vi "3D_Traverse_move.vi"(0 "Mode":T4=enum."Read traverse position", 1 "Route Checking?":bool=TRUE, 2 "Row Number":i32=-1, 5 "Position":sgl[](array[numeric])=[0.0, 0.0, 0.0] format="%#.2f", 7 "Work in Tunnel Coordinates":T2, 9 "Home":T1, 11 "Simulate/Run":T3=enum."Run VI", 12 "Traverse name":string, 13 "Backlash Compensation?":bool=TRUE, 14 "Currently on Point":i32=-1) -> (3 "Model  Roll        Pitch       Yaw (deg)":sgl[](array[numeric]) format="%#.2f", 4 "Trav Position achieved":sgl[](array[numeric]) format="%#.2f", 15 "Error String":string)   [LabVIEW 2014]
uses:
  Trav_mode.ctl
  Controls/User_Specific_mode.ctl
  Controls/Tunnel_Coordinates.ctl
  Controls/Home.ctl
  Controls/Global_mode.ctl
  Route mapping/Route_Display_Mode.ctl
  ADAM Client/Sub VIs/ADAM Controls/Update_scan_value.ctl
  Controls/In_Range.ctl
  Globals/Trav_pos_global.vi
  Globals/Preference_global.vi
  Globals/Constants_global.vi
  Route mapping/Route_mapping_global.vi
panel:
  in  "Position Increment":sgl[](array[numeric])=[0.0, 0.0, 0.0] step=1 format="%#.2f"
  out "Traverses Available":string[](array[string])
  in  "Traverse":u16(ring) items=["EnFlo_Measure_Height", "EnFlo_Stack", "EnFlo_Stack  dfg", "EnFlo_Trav3", "EnFlo_Tunnel", "EnFlo_Turntable"]
  # "X                Y                   Z"
  # "X                Y                   Z"
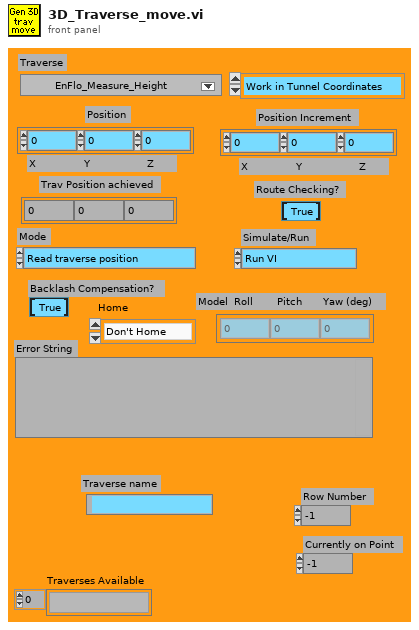
[diagram p1: front panel]
types:
  T1 = typedef "Home.ctl" = enum16{"Don't Home", "Home  +X", "Home  -X", "Home  +Y", "Home  -Y", "Home  +Z", "Home  -Z"}
  T2 = typedef "Tunnel_Coordinates.ctl" = enum16{"Work in Tunnel Coordinates", "Work in Model Coordinates"}
  T3 = typedef "User_Specific_mode.ctl" = enum16{"Check VI only", "Run VI"}
  T4 = typedef "Trav_mode.ctl" = enum16{"Move traverse", "Read traverse position", "Teach Position"}
  T5 = typedef "Global_mode.ctl" = enum16{"Read Global", "Load Global From File", "Write Global to File"}
  T6 = enum16{"To Traverse Coordinates", "To User Coordinates"}
  T7 = typedef "Route_Display_Mode.ctl" = enum16{"Display View Always", "Display View on Crash"}
  T8 = typedef "Update_scan_value.ctl" = cluster{"Channel Name":string, "New Value":dbl}
  T9 = typedef "In_Range.ctl" = enum16{"%", "±", "% & ±"}
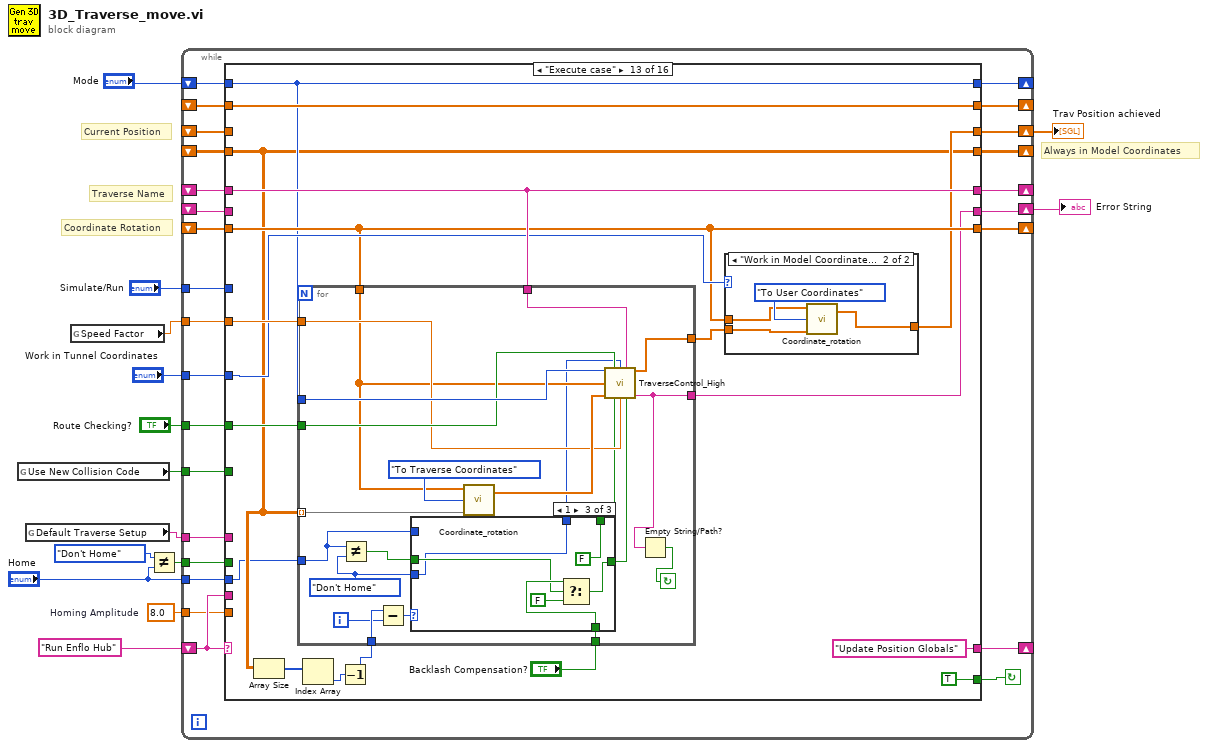
[diagram p0: block diagram]
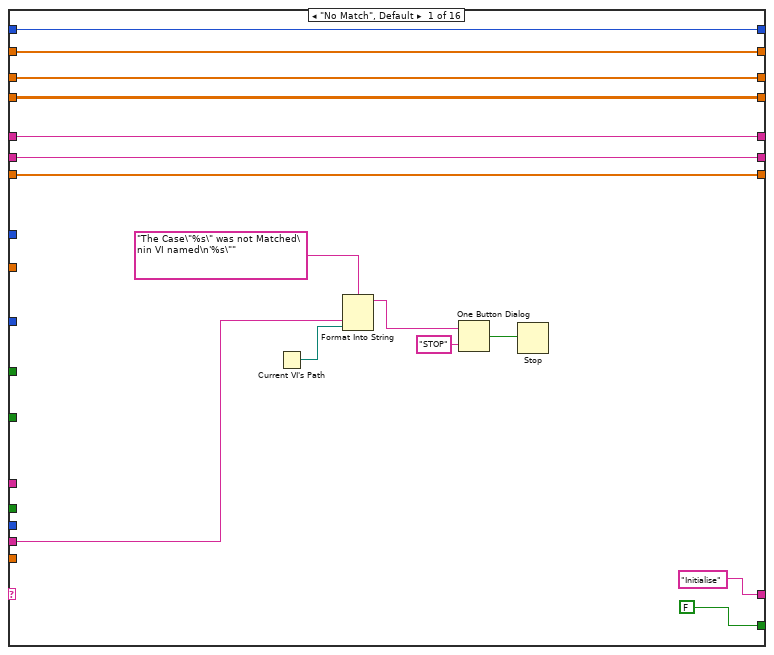
[diagram p2: hidden frame]
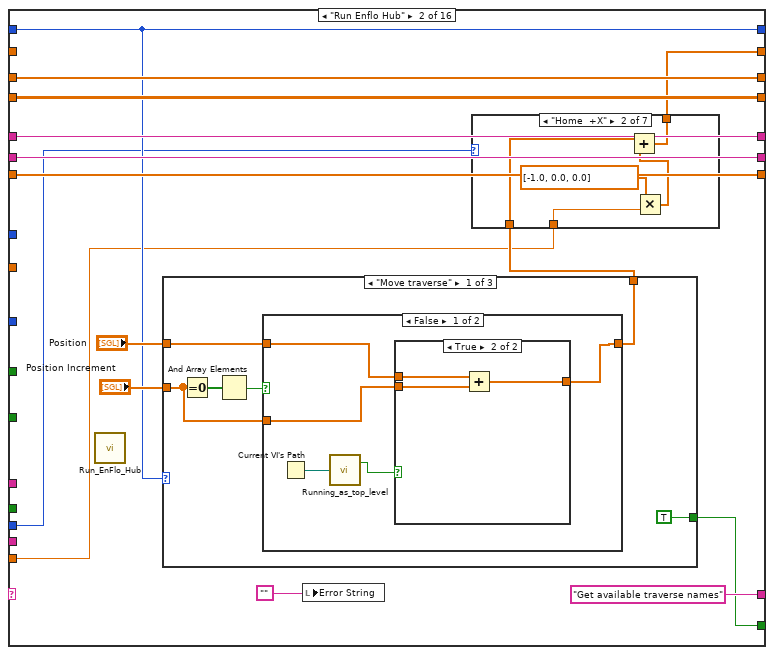
[diagram p3: hidden frame]
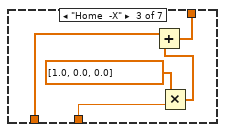
[diagram p5: hidden frame]
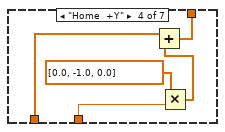
[diagram p6: hidden frame]
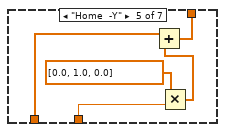
[diagram p7: hidden frame]
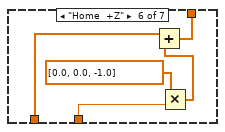
[diagram p8: hidden frame]
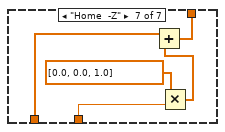
[diagram p9: hidden frame]
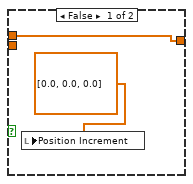
[diagram p10: hidden frame]
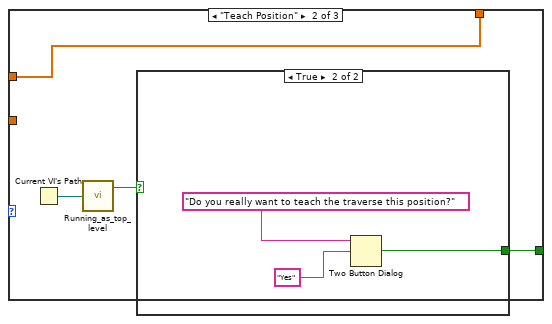
[diagram p12: hidden frame]
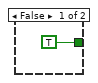
[diagram p13: hidden frame]
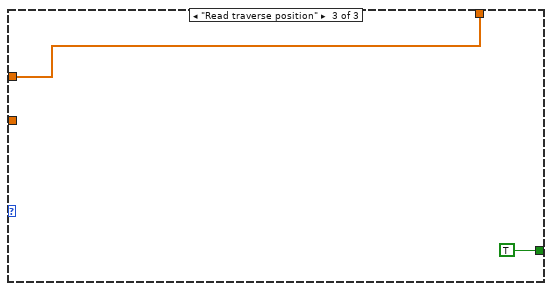
[diagram p14: hidden frame]
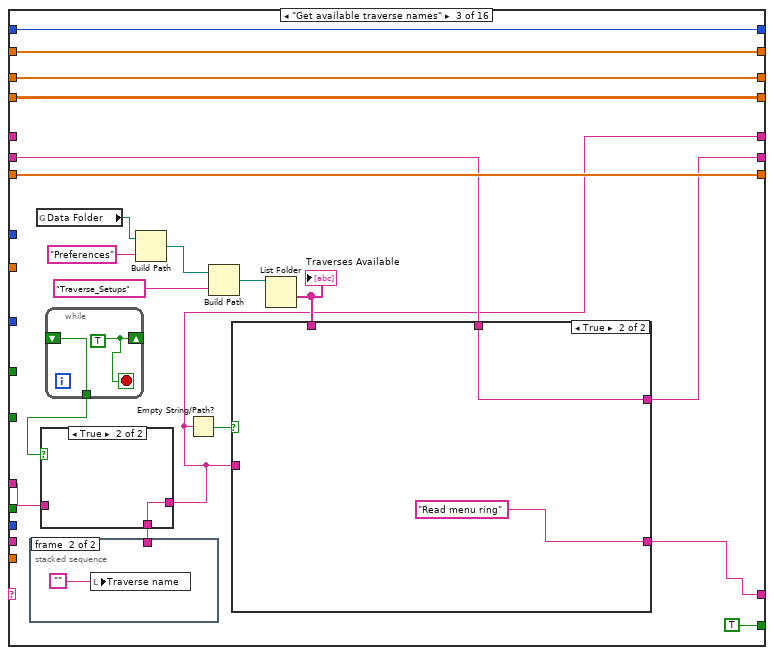
[diagram p15: hidden frame]
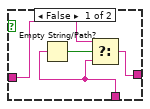
[diagram p16: hidden frame]
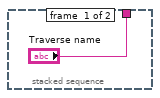
[diagram p17: hidden frame]
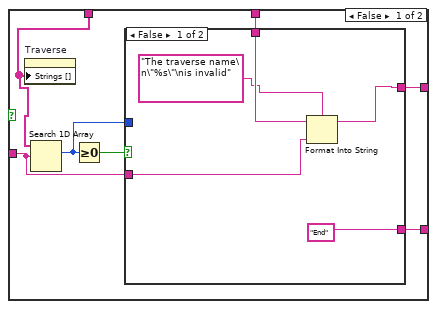
[diagram p18: hidden frame]
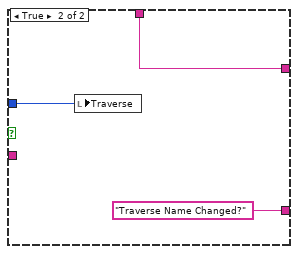
[diagram p19: hidden frame]
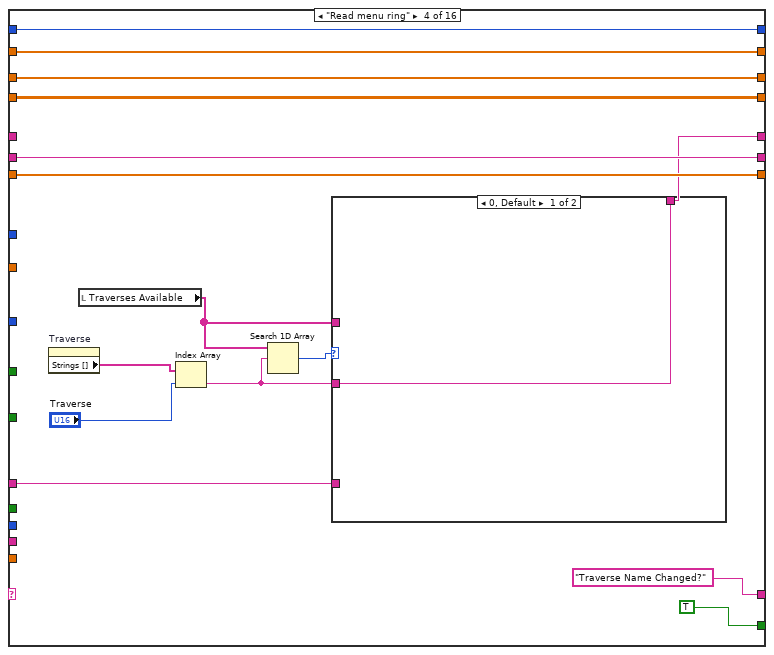
[diagram p20: hidden frame]
diagram:
  w5 = sgl 8.0  # Homing Amplitude
  # "Always in Model Coordinates"
  # "Current Position"
  # "Coordinate Rotation"
  # "Traverse Name"
  n1 = global read "Preference_global.vi" "Use New Collision Code"() -> (w1:bool)
  n2 = global read "Trav_pos_global.vi" "Default Traverse Setup"() -> (w7:string)
  n3 = global read "Trav_pos_global.vi" "Speed Factor"() -> (w11:sgl)
  n4 = Not Equal?(x=Home."Don't Home" ("Home"), y="Home") -> (x != y?=w2:bool)
  n5 = while {
    shift-left: "Run Enflo Hub" -> [w38]
    shift-right: [w39] -> _
    shift-right: [w36] -> _
    shift-left: _ -> [w34]
    tunnel: "Simulate/Run" -> [w37]
    shift-right: [w35] -> w12
    shift-left: _ -> [w33]
    shift-right: [w31] -> _
    shift-left: _ -> [w32]
    shift-right: [w28] -> _
    shift-left: _ -> [w27]
    shift-right: [w29] -> w8
    shift-left: _ -> [w30]
    tunnel: w11 -> [w26]
    tunnel: "Work in Tunnel Coordinates" -> [w25]
    tunnel: "Route Checking?" -> [w24]
    tunnel: w7 -> [w23]
    shift-right: [w22] -> _
    shift-left: _ -> [w21]
    shift-right: [w19] -> _
    shift-left: "Mode" -> [w20]
    tunnel: "Home" -> [w18]
    tunnel: w5 -> [w17]
    tunnel: w2 -> [w16]
    tunnel: w1 -> [w15]
    stop <- w40 continue-if-true
    n6 = case shown="\"Execute case\"" w38 {
      tunnel: [FALSE w63 TRUE TRUE TRUE TRUE w311 TRUE ("T button?") TRUE ("T button?") TRUE w503 w531 TRUE TRUE TRUE FALSE] -> w40
      tunnel: ["Initialise" "Get available traverse names" w139 "Traverse Name Changed?" "Mode" w261 w301 "Perform Route Check" w361 w403 "Display Traverse Views" w538 "Update Position Globals" "Tidy up" "End" "End"] -> w39
      tunnel: w38 -> [w50 _ _ _ _ _ _ _ _ _ _ _ _ _ _ _]
      tunnel: w37 -> [_ _ _ _ w214 w262 w306 _ w358 w399 _ w536 _ w626 w679 w776]
      tunnel: [w47 w69 w131 w175 w207 w253 w313 w338 w360 w398 w508 w543 w580 w625 w684 w772] -> w36
      tunnel: [w46 w68 w137 w187 "" w263 w312 "" w353 w407 w500 w540 w564 w629 w686 w779] -> w35
      tunnel: w34 -> [w47 w69 _ _ w207 w253 w313 w338 w360 w398 w508 w543 w580 w625 w684 w772]
      tunnel: w33 -> [w46 w68 w136 w187 _ w263 _ _ w355 _ w501 w540 _ w629 w687 w779]
      tunnel: w32 -> [w45 w67 w148 w186 _ w264 w309 w341 w356 w390 w496 w546 w577 w622 w689 w773]
      tunnel: [w45 w67 w148 w186 w206 w264 w309 w341 w356 w390 w496 w546 w577 w622 w689 w773] -> w31
      tunnel: w30 -> [w44 w66 w147 w185 w217 w255 w307 _ w352 w405 w507 w545 _ w624 w688 w774]
      tunnel: [w44 w66 w147 w185 w217 w255 w299 w340 w352 w406 w507 w545 w575 w624 w688 w774] -> w29
      tunnel: [w43 w65 w146 w184 w218 w265 w314 w344 w365 w393 w506 w544 w569 w630 w690 w780] -> w28
      tunnel: w27 -> [w43 w65 w146 w184 _ w265 w314 w344 w365 _ w506 w544 w569 w630 w690 w780]
      tunnel: w26 -> [_ _ _ _ _ _ _ _ _ _ _ _ w579 _ _ _]
      tunnel: w25 -> [_ _ _ _ w213 w257 w310 w342 w357 w408 w497 _ w578 w623 _ w775]
      tunnel: w24 -> [_ _ _ _ _ w258 _ _ _ _ _ _ w573 _ _ _]
      tunnel: w23 -> [_ _ w130 w179 _ _ _ _ _ _ _ _ _ _ _ _]
      tunnel: [w42 w58 w134 w177 w212 w254 w300 w339 w359 w397 w499 w530 w572 w628 w683 w777] -> w22
      tunnel: w21 -> [w42 _ w134 w177 w212 w254 w300 w339 w359 w397 w499 w530 w572 w628 w683 w777]
      tunnel: w20 -> [w41 w60 w133 w176 w208 w252 w298 w334 w366 w396 w498 w529 w571 w627 w682 w771]
      tunnel: [w41 w60 w133 w176 w209 w252 w298 w334 w366 w396 w498 w529 w571 w627 w682 w771] -> w19
      tunnel: w18 -> [_ w57 _ _ _ _ _ _ _ w395 _ _ w565 _ w681 _]
      tunnel: w17 -> [_ w56 _ _ _ _ _ _ _ w392 _ _ _ _ w680 _]
      tunnel: w16 -> [_ _ _ _ _ _ _ _ _ _ _ _ _ _ w678 _]
      tunnel: w15 -> [_ _ _ _ w196 _ _ _ _ w391 _ _ _ _ _ _]
      frame "No Match", Default {
        n7 = Current VI's Path() -> (path=w49:path)
        n8 = Format Into String(format string="The Case\"%s\" was not Matched\nin VI named\n'%s\"" ("Format String"), w50, w49) -> (resulting string=w53:string)  [unwired: 2 in, 1 out]
        n9 = One Button Dialog(message=w53, button name ("OK")="STOP") -> (true=w51:bool)
        n10 = Stop(stop? (T)=w51) -> ()
      }
      frame "Run Enflo Hub" {
        n11 = call "Run_EnFlo_Hub.vi"() -> ()  [unwired: 8 out]
        n12 = case shown="\"Move traverse\"" w60 {
          tunnel: [TRUE ("T button?") w120 TRUE ("T button?")] -> w63
          tunnel: [w104 w119 w128] -> w59
          tunnel: "Position" -> [w103 w119 w128]
          tunnel: "Position Increment" -> [w102 _ _]
          frame "Move traverse" {
            n13 = Equal To 0?(x=w102) -> (x = 0?=w106:bool[])
            n14 = And Array Elements(Boolean array=w106) -> (logical AND=w105:bool)
            n15 = case shown="False" w105 {
              tunnel: [w108 w118] -> w104
              tunnel: w103 -> [w110 w118]
              tunnel: w102 -> [w109 _]
              frame False {
                n16 = Current VI's Path() -> (path=w112:path)
                n17 = call "Running_as_top_level.vi"("Vi path name"=w112) -> ("Top Level"=w111:bool)  [unwired: 1 out]
                n18 = case shown="True" w111 {
                  tunnel: w110 -> [w114 w117]
                  tunnel: w109 -> [_ w116]
                  tunnel: [w114 w115] -> w108
                  frame False {
                    n19 = local write "Position Increment"(sgl[] [0.0, 0.0, 0.0] ("Position Increment")) -> ()
                  }
                  frame True {
                    n20 = Add(x=w117, y=w116) -> (x+y=w115:sgl[])
                  }
                }
              }
              frame True {
              }
            }
          }
          frame "Teach Position" {
            n21 = Current VI's Path() -> (path=w122:path)
            n22 = call "Running_as_top_level.vi"("Vi path name"=w122) -> ("Top Level"=w121:bool)  [unwired: 1 out]
            n23 = case shown="True" w121 {
              tunnel: [TRUE ("T button?") w124] -> w120
              frame False {
              }
              frame True {
                n24 = Two Button Dialog(message="Do you really want to teach the traverse this position?", 2:"Yes" ("T button name (\"OK\")")) -> (T button?=w124:bool)  [unwired: 1 out]
              }
            }
          }
          frame "Read traverse position" {
          }
        }
        n25 = local write "Error String"("") -> ()
        n26 = case shown="\"Home  +X\"" w57 {
          tunnel: [w71 w75 w80 w85 w90 w95 w100] -> w58
          tunnel: w59 -> [w71 w76 w81 w86 w91 w96 w101]
          tunnel: w56 -> [_ w72 w77 w82 w87 w92 w97]
          frame "Don't Home" {
          }
          frame "Home  +X" {
            n27 = Multiply(x=sgl[] [-1.0, 0.0, 0.0] ("y"), y=w72) -> (x*y=w73:sgl[])
            n28 = Add(x=w76, y=w73) -> (x+y=w75:sgl[])
          }
          frame "Home  -X" {
            n29 = Multiply(x=sgl[] [1.0, 0.0, 0.0] ("y"), y=w77) -> (x*y=w78:sgl[])
            n30 = Add(x=w81, y=w78) -> (x+y=w80:sgl[])
          }
          frame "Home  +Y" {
            n31 = Multiply(x=sgl[] [0.0, -1.0, 0.0] ("y"), y=w82) -> (x*y=w83:sgl[])
            n32 = Add(x=w86, y=w83) -> (x+y=w85:sgl[])
          }
          frame "Home  -Y" {
            n33 = Multiply(x=sgl[] [0.0, 1.0, 0.0] ("y"), y=w87) -> (x*y=w88:sgl[])
            n34 = Add(x=w91, y=w88) -> (x+y=w90:sgl[])
          }
          frame "Home  +Z" {
            n35 = Multiply(x=sgl[] [0.0, 0.0, -1.0] ("y"), y=w92) -> (x*y=w93:sgl[])
            n36 = Add(x=w96, y=w93) -> (x+y=w95:sgl[])
          }
          frame "Home  -Z" {
            n37 = Multiply(x=sgl[] [0.0, 0.0, 1.0] ("y"), y=w97) -> (x*y=w98:sgl[])
            n38 = Add(x=w101, y=w98) -> (x+y=w100:sgl[])
          }
        }
      }
      frame "Get available traverse names" {
        n39 = stacked-sequence {
          tunnel: ["Traverse name" _] -> w129
          frame #0 {
          }
          frame #1 {
            n40 = local write "Traverse name"("") -> ()
          }
        }
        n41 = global read "Constants_global.vi" "Data Folder"() -> (w142:path)
        n42 = while {
          shift-right: [w156] -> _
          shift-left: _ -> [w157]
          tunnel: [w157] -> w132
          stop <- w156 stop-if-true
          w156 = TRUE
        }
        n43 = case shown="True" w132 {
          tunnel: [w151 w153] -> w131
          tunnel: w130 -> [w150 _]
          tunnel: w129 -> [w149 w153]
          frame False {
            n44 = Empty String/Path?(string/path=w149) -> (empty?=w152:bool)
            n45 = Select(t=w150, s=w152, f=w149) -> (s? t:f=w151:string)
          }
          frame True {
          }
        }
        n46 = Build Path(base path=w142, name or relative path="Preferences") -> (appended path=w144:path)
        n47 = Empty String/Path?(string/path=w131) -> (empty?=w140:bool)
        n48 = Build Path(base path=w144, name or relative path="Traverse_Setups") -> (appended path=w145:path)
        n49 = List Folder(path=w145) -> (folder names=w138:string[])  [unwired: 1 in, 5 out]
        "Traverses Available" <- w138
        n50 = case shown="True" w140 {
          tunnel: [w161 "Read menu ring"] -> w139
          tunnel: w138 -> [w158 _]
          tunnel: w131 -> [w164 _]
          tunnel: [w163 w173] -> w137
          tunnel: w136 -> [w162 w173]
          frame False {
            n51 = property on="Traverse" class="Ring (strict)"("Strings []"=w158) -> ()  [unwired: 2 in, 2 out]
            n52 = Search 1D Array(1D array=w158, element=w164) -> (index of element=w159:i32)  [unwired: 1 out]
            n53 = Greater Or Equal To 0?(x=w159) -> (x >= 0?=w160:bool)
            n54 = case shown="False" w160 {
              tunnel: w164 -> [w169 _]
              tunnel: [w166 w172] -> w163
              tunnel: w162 -> [w168 w172]
              tunnel: ["End" "Traverse Name Changed?"] -> w161
              tunnel: w159 -> [_ w170]
              frame False {
                n55 = Format Into String(format string="The traverse name\n\"%s\"\nis invalid", initial string=w168, w169) -> (resulting string=w166:string)  [unwired: 1 in, 1 out]
              }
              frame True {
                n56 = local write "Traverse"(w170) -> ()
              }
            }
          }
          frame True {
          }
        }
      }
      frame "Read menu ring" {
        n57 = property on="Traverse" class="Ring (strict)"() -> ("Strings []"=w183:string[])  [unwired: 2 in, 2 out]
        n58 = local read "Traverses Available"() -> (w180:string[])
        n59 = Index Array(array=w183, index="Traverse") -> (element=w178:string)
        n60 = Search 1D Array(1D array=w180, element=w178) -> (index of element=w181:i32)  [unwired: 1 out]
        n61 = case shown="0, Default" w181 {
          tunnel: w180 -> [_ w193]
          tunnel: w179 -> [_ w191]
          tunnel: [w190 w191] -> w175
          tunnel: w178 -> [w190 _]
          frame 0, Default {
          }
          frame -1 {
            n62 = property on="Traverse" class="Ring (strict)"("Strings []"=w193) -> ()  [unwired: 2 in, 2 out]
            n63 = Search 1D Array(1D array=w193, element=w191) -> (index of element=w192:i32)  [unwired: 1 out]
            n64 = local write "Traverse"(w192) -> ()
          }
        }
      }
      frame "Traverse Name Changed?" {
        n65 = call "Rig_Pict_Display_Pref.vi"("Traverse Name"=w207) -> ("Roll Pitch Yaw ADAM Channels"=w205:string[])  [unwired: 3 in, 4 out]
        n66 = Build Array (concatenate)(w205, "EnFlo_Tunnel:Trav Origin:X Offset") -> (w203:string[])
        n67 = case shown="\"Run VI\"" w214 {
          tunnel: [w234 w245] -> w195
          tunnel: w203 -> [w236 w246]
          frame "Check VI only" {
            n68 = call "Read_Write_Local_table.vi"("Mode"=Global_mode."Read Global") -> ("Ch Names"=w237:string[], "Ch Values Out"=w235:T8[])  [unwired: 2 in, 1 out]
            n69 = for {
              tunnel: w237 -> [w244]
              tunnel: w236 -> [w243] mode=indexing
              tunnel: w235 -> [w242]
              tunnel: [w239] -> w234 mode=indexing
              n70 = Search 1D Array(1D array=w244, element=w243) -> (index of element=w241:i32)  [unwired: 1 out]
              n71 = Index Array(array=w242, index=w241) -> (element=w240:T8)
              n72 = Unbundle By Name(w240) -> ("New Value"=w239:dbl)
            }
          }
          frame "Run VI" {
            n73 = call "Get_Current_Scan_client.vi"("ADAM Ch Names"=w246) -> ("Numerical Values"=w245:dbl[])  [unwired: 3 out]
          }
        }
        n74 = Build Array(TRUE) -> ()  [unwired: 1 out]
        n75 = To Single Precision Float(number=w195) -> (single precision float=w194:sgl[])
        n76 = Split 1D Array(array=w194, index=3) -> (first subarray=w201:sgl[], second subarray=w199:sgl[])
        n77 = global read "Route_mapping_global.vi" "Traverse Setup"() -> (w197:string)
        n78 = for {
          tunnel: w201 -> [w232] mode=indexing
          tunnel: [w230] -> w206 mode=indexing
          n79 = Not A Number/Path/Refnum?(number/path/refnum=w232) -> (NaN/Path/Refnum?=w233:bool)
          n80 = Select(t=sgl 0.0, s=w233, f=w232) -> (s? t:f=w230:sgl)
        }
        "Model  Roll        Pitch       Yaw (deg)" <- w206
        n81 = case shown="\"Work in Tunnel Coordinates\"" w213 {
          tunnel: w212 -> [w249 w251]
          tunnel: [w248 w251] -> w215
          tunnel: w206 -> [w247 _]
          frame "Work in Tunnel Coordinates" {
            n82 = call "Coordinate_rotation.vi"("Model       Roll      Pitch       Yaw (deg)"=w247, "Input Position"=w249, "Mode"=T6."To User Coordinates") -> ("Output Position"=w248:sgl[])  [unwired: 2 in, 1 out]
          }
          frame "Work in Model Coordinates" {
          }
        }
        n83 = Build Array(w215) -> (w218:sgl[][])
        n84 = Index Array(array=w199) -> (element=w200:sgl)  [unwired: 1 in]
        n85 = global write "Trav_pos_global.vi" "Traverse Origin X Offset (mm)"(w200) -> ()
        n86 = Equal?(x=w197, y=w207) -> (x = y?=w198:bool)
        n87 = case shown="False" w198 {
          tunnel: w207 -> [w225 _]
          tunnel: [w223 FALSE ("Top Level")] -> w211
          tunnel: w196 -> [w222 _]
          frame False {
            n88 = Current VI's Path() -> (path=w224:path)
            n89 = call "Running_as_top_level.vi"("Vi path name"=w224) -> ("Top Level"=w223:bool)  [unwired: 1 out]
            n90 = case shown="True" w222 {
              tunnel: w225 -> [w226 w228]
              frame False {
                w227 = FALSE  # Show Panel?
                n91 = call "Traverse_Space.vi"("Show Panel?"=w227, "Traverse Setup"=w226) -> ()  [unwired: 1 in, 8 out]
              }
              frame True {
                n92 = global write "Route_mapping_global.vi" "Traverse Setup"(w228) -> ()
              }
            }
          }
          frame True {
          }
        }
        n93 = Select(t=Trav_mode."Read traverse position" ("Mode"), s=w211, f=w208) -> (s? t:f=w209:T4)
      }
      frame "Mode" {
        n94 = while {
          shift-right: [w269] -> _
          shift-left: _ -> [w268]
          tunnel: w257 -> [w269]
          tunnel: [w267] -> w256
          stop <- TRUE stop-if-true
          n95 = Equal?(x=w268, y=w269) -> (x = y?=w267:bool)
        }
        n96 = case shown="\"Run VI\"" w262 {
          tunnel: w252 -> [_ w277]
          tunnel: [w271 w276] -> w261
          tunnel: "Execute case" -> [_ w275]
          tunnel: "Read Current Position" -> [w271 w274]
          tunnel: w258 -> [_ w273]
          tunnel: w256 -> [_ _]
          tunnel: w253 -> [_ w272]
          frame "Check VI only" {
          }
          frame "Run VI" {
            n97 = case shown="\"Move traverse\"" w277 {
              tunnel: [w280 w297] -> w276
              tunnel: w275 -> [w279 w297]
              tunnel: w274 -> [w278 _]
              tunnel: w273 -> [w281 _]
              tunnel: w272 -> [w282 _]
              frame "Move traverse" {
                n98 = case shown="True" w281 {
                  tunnel: w282 -> [_ w293]
                  tunnel: [w283 w287] -> w280
                  tunnel: w279 -> [w283 _]
                  tunnel: w278 -> [_ w285]
                  frame False {
                  }
                  frame True {
                    n99 = global read "Constants_global.vi" "Traverse folder"() -> (w294:path)
                    n100 = Build Path(base path=w294, name or relative path=w293) -> (appended path=w296:path)
                    n101 = Build Path(base path=w296, name or relative path="Traverse_Pos.xls" ("Substring")) -> (appended path=w292:path)
                    n102 = File/Directory Info(path=w292) -> (last mod=w290:timestamp)  [unwired: 1 in, 6 out]
                    n103 = Get Date/Time In Seconds() -> (seconds since 1Jan1904=w291:timestamp)
                    n104 = Subtract(x=w291, y=w290) -> (x-y=w289:dbl)
                    n105 = Greater?(x=w289, y=40.0) -> (0:w286:bool)
                    n106 = Select(t=w285, s=w286, f="Quick Read from file") -> (s? t:f=w287:string)
                  }
                }
              }
              frame "Read traverse position", Default {
              }
            }
          }
        }
      }
      frame "Read Current Position" {
        n107 = case shown="\"Run VI\"" w306 {
          tunnel: w313 -> [w315 w326]
          tunnel: ["" w328] -> w312
          tunnel: w309 -> [_ w322]
          tunnel: [w316 w327] -> w308
          tunnel: w307 -> [_ w321]
          frame "Check VI only" {
            n108 = call "Read-Write_Check_Pos.vi"("Mode"=enum16{"Read", "Write"}."Read", "Traverse Name"=w315) -> ("Position Output"=w316:sgl[])  [unwired: 1 in]
          }
          frame "Run VI" {
            w320 = TRUE  # Last Part of Move?
            w325 = FALSE  # Route Checking?
            w324 = FALSE  # Backlash Compensation?
            n109 = call "TraverseControl_High.vi"("Mode"=Trav_mode."Read traverse position", "Route Checking?"=w325, "Home"=Home."Don't Home", "Traverse Name"=w326, "Model       Roll      Pitch       Yaw (deg)"=w322, "Position input XYZ"=w321, "Last Part of Move?"=w320, "Backlash Compensation?"=w324) -> ("Position Output XYZ"=w327:sgl[], "Error String"=w328:string)  [unwired: 6 in]
          }
        }
        n110 = Equal?(x=Trav_mode."Read traverse position" ("Mode"), y=w298) -> (x = y?=w304:bool)
        n111 = case shown="\"Work in Tunnel Coordinates\"" w310 {
          tunnel: w308 -> [w329 w331]
          tunnel: [w329 w332] -> w299
          tunnel: w309 -> [_ w330]
          frame "Work in Tunnel Coordinates" {
          }
          frame "Work in Model Coordinates" {
            n112 = call "Coordinate_rotation.vi"("Model       Roll      Pitch       Yaw (deg)"=w330, "Input Position"=w331, "Mode"=T6."To User Coordinates") -> ("Output Position"=w332:sgl[])  [unwired: 2 in, 1 out]
          }
        }
        n113 = Empty String/Path?(string/path=w312) -> (empty?=w311:bool)
        n114 = Select(t="Update Position Globals", s=w304, f="Perform Route Check") -> (s? t:f=w301:string)
      }
      frame "Quick Read from file" {
        n115 = call "Read_Traverse_Pos_File.vi"("Traverse Name"=w338) -> ("Tunnel Coordinates"=w337:sgl[])
        n116 = case shown="\"Work in Model Coordinates\"" w342 {
          tunnel: w337 -> [w345 w348]
          tunnel: [w345 w347] -> w340
          tunnel: w341 -> [_ w346]
          frame "Work in Tunnel Coordinates" {
          }
          frame "Work in Model Coordinates" {
            n117 = call "Coordinate_rotation.vi"("Model       Roll      Pitch       Yaw (deg)"=w346, "Input Position"=w348, "Mode"=T6."To User Coordinates") -> ("Output Position"=w347:sgl[])  [unwired: 2 in, 1 out]
          }
        }
      }
      frame "Perform Route Check" {
        n118 = for {
          N: 2 -> [_]
          tunnel: w360 -> [w375]
          tunnel: w359 -> [w374]
          tunnel: w358 -> [w373]
          tunnel: w357 -> [w372]
          tunnel: w356 -> [w371]
          tunnel: [w368] -> w354
          tunnel: w352 -> [w370]
          tunnel: [w367] -> w350
          i -> [w369]
          stop <- w367 stop-if-true
          n119 = case shown="0, Default" w369 {
            tunnel: w375 -> [w382 w389]
            tunnel: w374 -> [w381 w388]
            tunnel: w373 -> [w380 w387]
            tunnel: w372 -> [w379 w386]
            tunnel: w371 -> [w378 w385]
            tunnel: [w377 w384] -> w368
            tunnel: w370 -> [w376 w383]
            frame 1 {
              n120 = call "Traverse_to_Traverse_Collision.vi"("Current Position"=w376, "Traverse Name"=w382, "Model  Roll        Pitch       Yaw (deg)"=w378, "Work in Tunnel Coordinates"=w379, "Simulate/Run"=w380, "New Position"=w381) -> ("Error String"=w377:string)  [unwired: 5 in]
            }
            frame 0, Default {
              n121 = call "Traverse_to_Traverse_Collision.vi"("Current Position"=w383, "Traverse Name"=w389, "Model  Roll        Pitch       Yaw (deg)"=w385, "Work in Tunnel Coordinates"=w386, "Simulate/Run"=w387, "New Position"=w388) -> ("Error String"=w384:string)  [unwired: 5 in]
            }
          }
          n122 = Empty String/Path?(string/path=w368) -> (empty?=w367:bool)
        }
        n123 = Select(t="Perform Route Check_2" ("f"), s=w350, f="Route Error") -> (s? t:f=w361:string)
        n124 = Concatenate Strings(w355, w354) -> (w353:string)
      }
      frame "Perform Route Check_2" {
        n125 = case shown="True" w391 {
          tunnel: w408 -> [w418 w436]
          tunnel: [w409 w434] -> w407
          tunnel: w405 -> [w417 w433]
          tunnel: w399 -> [w412 w432]
          tunnel: w398 -> [w413 w431]
          tunnel: w397 -> [w416 w430]
          tunnel: [w410 w428] -> w394
          tunnel: w390 -> [w411 w427]
          frame True {
            n126 = case shown="\"Work in Tunnel Coordinates\"" w418 {
              tunnel: w411 -> [_ w425]
              tunnel: w416 -> [w419 w421]
              tunnel: w417 -> [w420 w424]
              tunnel: [w419 w423] -> w414
              tunnel: [w420 w422] -> w415
              frame "Work in Tunnel Coordinates" {
              }
              frame "Work in Model Coordinates" {
                w426 = T6."To Traverse Coordinates" ("Mode")
                n127 = call "Coordinate_rotation.vi"("Model       Roll      Pitch       Yaw (deg)"=w425, "Input Position"=w424, "Mode"=w426) -> ("Output Position"=w422:sgl[])  [unwired: 2 in, 1 out]
                n128 = call "Coordinate_rotation.vi"("Model       Roll      Pitch       Yaw (deg)"=w425, "Input Position"=w421, "Mode"=w426) -> ("Output Position"=w423:sgl[])  [unwired: 2 in, 1 out]
              }
            }
            n129 = call "Check_with_Jump_PN.vi"("Current position"=w415, "Traverse Name"=w413, "Simulate/Run"=w412, "New Position"=w414, "Model       Roll      Pitch       Yaw (deg)"=w411) -> ("Error Comments"=w409:string, "Steps"=w410:dbl[][])  [unwired: 9 in]
          }
          frame False {
            n130 = case shown="\"Work in Model Coordinates\"" w436 {
              tunnel: w427 -> [w441 _]
              tunnel: w430 -> [w437 w443]
              tunnel: w433 -> [w440 w444]
              tunnel: [w439 w443] -> w429
              tunnel: [w438 w444] -> w435
              frame "Work in Tunnel Coordinates" {
                w442 = T6."To User Coordinates" ("Mode")
                n131 = call "Coordinate_rotation.vi"("Model       Roll      Pitch       Yaw (deg)"=w441, "Input Position"=w440, "Mode"=w442) -> ("Output Position"=w438:sgl[])  [unwired: 2 in, 1 out]
                n132 = call "Coordinate_rotation.vi"("Model       Roll      Pitch       Yaw (deg)"=w441, "Input Position"=w437, "Mode"=w442) -> ("Output Position"=w439:sgl[])  [unwired: 2 in, 1 out]
              }
              frame "Work in Model Coordinates" {
              }
            }
            n133 = call "Check_with_Jump.vi"("Current position"=w435, "Traverse Name"=w431, "Simulate/Run"=w432, "New Position"=w429, "Model       Roll      Pitch       Yaw (deg)"=w427) -> ("Error Comments"=w434:string, "Steps"=w428:sgl[][])  [unwired: 9 in]
          }
        }
        n134 = case shown="\"Don't Home\"" w395 {
          tunnel: w394 -> [w445 w452 w460 w468 w476 w484 w492]
          tunnel: [w445 w451 w459 w467 w475 w483 w491] -> w393
          tunnel: w392 -> [_ w446 w454 w462 w470 w478 w486]
          frame "Don't Home" {
          }
          frame "Home  +X" {
            n135 = for {
              tunnel: [w453] -> w450
              tunnel: w452 -> [w453] mode=indexing
            }
            n136 = Multiply(x=dbl[] [2.0, 0.0, 0.0] ("y"), y=w446) -> (x*y=w447:dbl[])
            n137 = Add(x=w450, y=w447) -> (x+y=w449:dbl[])
            n138 = Build Array (concatenate)(w452, w449) -> (w451:dbl[][])
          }
          frame "Home  -X" {
            n139 = for {
              tunnel: [w461] -> w458
              tunnel: w460 -> [w461] mode=indexing
            }
            n140 = Multiply(x=dbl[] [-2.0, 0.0, 0.0] ("y"), y=w454) -> (x*y=w455:dbl[])
            n141 = Add(x=w458, y=w455) -> (x+y=w457:dbl[])
            n142 = Build Array (concatenate)(w460, w457) -> (w459:dbl[][])
          }
          frame "Home  +Y" {
            n143 = for {
              tunnel: [w469] -> w466
              tunnel: w468 -> [w469] mode=indexing
            }
            n144 = Multiply(x=dbl[] [0.0, 2.0, 0.0] ("y"), y=w462) -> (x*y=w463:dbl[])
            n145 = Add(x=w466, y=w463) -> (x+y=w465:dbl[])
            n146 = Build Array (concatenate)(w468, w465) -> (w467:dbl[][])
          }
          frame "Home  -Y" {
            n147 = for {
              tunnel: [w477] -> w474
              tunnel: w476 -> [w477] mode=indexing
            }
            n148 = Multiply(x=dbl[] [0.0, -2.0, 0.0] ("y"), y=w470) -> (x*y=w471:dbl[])
            n149 = Add(x=w474, y=w471) -> (x+y=w473:dbl[])
            n150 = Build Array (concatenate)(w476, w473) -> (w475:dbl[][])
          }
          frame "Home  +Z" {
            n151 = for {
              tunnel: [w485] -> w482
              tunnel: w484 -> [w485] mode=indexing
            }
            n152 = Multiply(x=dbl[] [0.0, 0.0, 2.0] ("y"), y=w478) -> (x*y=w479:dbl[])
            n153 = Add(x=w482, y=w479) -> (x+y=w481:dbl[])
            n154 = Build Array (concatenate)(w484, w481) -> (w483:dbl[][])
          }
          frame "Home  -Z" {
            n155 = for {
              tunnel: [w493] -> w490
              tunnel: w492 -> [w493] mode=indexing
            }
            n156 = Multiply(x=dbl[] [0.0, 0.0, -2.0] ("y"), y=w486) -> (x*y=w487:dbl[])
            n157 = Add(x=w490, y=w487) -> (x+y=w489:dbl[])
            n158 = Build Array (concatenate)(w492, w489) -> (w491:dbl[][])
          }
        }
        n159 = Empty String/Path?(string/path=w407) -> (empty?=w400:bool)
        n160 = case shown="True" w400 {
          tunnel: [w494 w495] -> w406
          tunnel: w405 -> [w494 _]
          tunnel: w397 -> [_ w495]
          frame False {
          }
          frame True {
          }
        }
        n161 = Select(t="Display Traverse Views", s=w400, f="Route Error") -> (s? t:f=w403:string)
      }
      frame "Route Error" {
        n162 = global read "Trav_pos_global.vi" "Jump Bad Positions?"() -> (w505:bool)
        n163 = case shown="True" w505 {
          tunnel: w499 -> [_ w513]
          tunnel: [TRUE w512] -> w503
          tunnel: w497 -> [_ w511]
          tunnel: w496 -> [_ w510]
          frame False {
          }
          frame True {
            n164 = Current VI's Path() -> (path=w515:path)
            n165 = call "Running_as_top_level.vi"("Vi path name"=w515) -> ("Top Level"=w514:bool)  [unwired: 1 out]
            n166 = case shown="False" w514 {
              tunnel: w513 -> [w517 _]
              tunnel: [FALSE TRUE] -> w512
              tunnel: w511 -> [w519 _]
              tunnel: w510 -> [w516 _]
              frame False {
                n167 = case shown="\"Work in Tunnel Coordinates\"" w519 {
                  tunnel: [w524 w527] -> w518
                  tunnel: w517 -> [w525 w527]
                  tunnel: w516 -> [w523 _]
                  frame "Work in Tunnel Coordinates" {
                    n168 = call "Coordinate_rotation.vi"("Model       Roll      Pitch       Yaw (deg)"=w523, "Input Position"=w525, "Mode"=T6."To User Coordinates") -> ("Output Position"=w524:sgl[])  [unwired: 2 in, 1 out]
                  }
                  frame "Work in Model Coordinates" {
                  }
                }
                n169 = global read "Trav_pos_global.vi" "Jumped Positions"() -> (w521:dbl[][])
                n170 = Build Array (concatenate)(w518, w521) -> (w520:dbl[][])
                n171 = global write "Trav_pos_global.vi" "Jumped Positions"(w520) -> ()
              }
              frame True {
              }
            }
          }
        }
        n172 = Concatenate Strings("Route Checking Error\n" ("string"), w501) -> (w500:string)
      }
      frame "Display Traverse Views" {
        n173 = global read "Route_mapping_global.vi" "Display Mode"() -> (w542:T7)
        n174 = Equal?(x=w536, y=User_Specific_mode."Check VI only" ("Simulate/Run")) -> (x = y?=w535:bool)
        n175 = Empty String/Path?(string/path=w540) -> (empty?=w531:bool)
        n176 = Equal?(x=w542, y=Route_Display_Mode."Display View Always" ("Display Mode")) -> (x = y?=w539:bool)
        n177 = Not(x=w531) -> (.not. x?=w532:bool)
        n178 = Or(x=w539, y=w532) -> (x .or. y?=w534:bool)
        n179 = And(x=w535, y=w534) -> (x .and. y?=w533:bool)
        n180 = case shown="True" w533 {
          tunnel: w544 -> [_ w555]
          tunnel: w543 -> [_ w554]
          tunnel: w540 -> [_ w551]
          tunnel: w531 -> [_ w549]
          frame False {
          }
          frame True {
            n181 = Not(x=w549) -> (.not. x?=w550:bool)
            n182 = for {
              tunnel: w555 -> [w562] mode=indexing
              tunnel: w554 -> [w561]
              tunnel: "Currently on Point" -> [w560]
              tunnel: "Row Number" -> [w559]
              tunnel: w551 -> [w558]
              tunnel: w550 -> [w556]
              n183 = Build Array(w562) -> (w563:dbl[][])
              n184 = call "Display_Trav_Views.vi"("Current Probe Position"=w563, "Traverse Name"=w561, "Currently on point"=w560, "Open Front Panel"=TRUE, "Error Comments"=w558, "Crash?"=w556, "Row Number"=w559) -> ()  [unwired: 4 out]
            }
          }
        }
        n185 = case shown="\"Check VI only\"" w536 {
          tunnel: ["Update Position Globals" "Execute case"] -> w538
          frame "Check VI only" {
          }
          frame "Run VI" {
          }
        }
      }
      frame "Execute case" {
        n186 = Array Size(array=w569) -> (size(s)=w570:i32[])
        n187 = Index Array(array=w570) -> (element=w568:i32)  [unwired: 1 in]
        n188 = Decrement(x=w568) -> (x-1=w567:i32)
        n189 = for {
          tunnel: w580 -> [w596]
          tunnel: w569 -> [w602] mode=indexing
          tunnel: w579 -> [w595]
          tunnel: w571 -> [w598]
          tunnel: w577 -> [w593]
          tunnel: [w600] -> w576
          tunnel: [w594] -> w564
          tunnel: w573 -> [w597]
          tunnel: w567 -> [w589]
          tunnel: w565 -> [w582]
          tunnel: "Backlash Compensation?" -> [w586]
          i -> [w588]
          stop <- w592 continue-if-true
          w583 = Home."Don't Home" ("Home")
          n190 = Not Equal?(x=w582, y=w583) -> (x != y?=w584:bool)
          n191 = Subtract(x=w589, y=w588) -> (x-y=w587:i32)
          n192 = case shown="1" w587 {
            tunnel: [w606 w610 w614] -> w591
            tunnel: [w603 w609 w611] -> w590
            tunnel: w586 -> [w608 _ w616]
            tunnel: [TRUE w610 FALSE ("f")] -> w585
            tunnel: w584 -> [w604 _ w612]
            tunnel: w583 -> [_ w609 w611]
            tunnel: w582 -> [w603 _ _]
            frame 0 {
              n193 = Select(t=FALSE, s=w604, f=w608) -> (s? t:f=w606:bool)
            }
            frame Default {
              w610 = FALSE ("f")
            }
            frame 1 {
              n194 = Select(t=w616, s=w612, f=FALSE) -> (s? t:f=w614:bool)
            }
          }
          n195 = call "Coordinate_rotation.vi"("Model       Roll      Pitch       Yaw (deg)"=w593, "Input Position"=w602, "Mode"=T6."To Traverse Coordinates") -> ("Output Position"=w599:sgl[])  [unwired: 2 in, 1 out]
          n196 = call "TraverseControl_High.vi"("Mode"=w598, "Route Checking?"=w597, "Home"=w590, "Traverse Name"=w596, "Model       Roll      Pitch       Yaw (deg)"=w593, "Position input XYZ"=w599, "Last Part of Move?"=w585, "Speed Factor"=w595, "Backlash Compensation?"=w591) -> ("Position Output XYZ"=w600:sgl[], "Error String"=w594:string)  [unwired: 5 in]
          n197 = Empty String/Path?(string/path=w594) -> (empty?=w592:bool)
        }
        n198 = case shown="\"Work in Model Coordinates\"" w578 {
          tunnel: w576 -> [w617 w620]
          tunnel: [w617 w619] -> w575
          tunnel: w577 -> [_ w618]
          frame "Work in Tunnel Coordinates" {
          }
          frame "Work in Model Coordinates" {
            n199 = call "Coordinate_rotation.vi"("Model       Roll      Pitch       Yaw (deg)"=w618, "Input Position"=w620, "Mode"=T6."To User Coordinates") -> ("Output Position"=w619:sgl[])  [unwired: 2 in, 1 out]
          }
        }
      }
      frame "Update Position Globals" {
        n200 = case shown="\"Run VI\"" w626 {
          tunnel: w625 -> [w636 _]
          tunnel: w624 -> [w635 _]
          tunnel: w623 -> [w634 _]
          tunnel: w622 -> [w633 _]
          frame "Check VI only" {
            n201 = stacked-sequence {
              seq-local: [w637 _] -> [_ w646]
              tunnel: w636 -> [_ w654]
              tunnel: w635 -> [w638 _]
              tunnel: w634 -> [w640 _]
              tunnel: w633 -> [w639 _]
              frame #0 {
                n202 = case shown="\"Work in Model Coordinates\"" w640 {
                  tunnel: w638 -> [w641 w644]
                  tunnel: [w641 w643] -> w637
                  tunnel: w639 -> [_ w642]
                  frame "Work in Tunnel Coordinates" {
                  }
                  frame "Work in Model Coordinates" {
                    n203 = call "Coordinate_rotation.vi"("Model       Roll      Pitch       Yaw (deg)"=w642, "Input Position"=w644, "Mode"=T6."To Traverse Coordinates") -> ("Output Position"=w643:sgl[])  [unwired: 2 in, 1 out]
                  }
                }
              }
              frame #1 {
                n204 = global read "Trav_pos_global.vi" "Route checking Chs"() -> (w653:string[])
                n205 = global read "Trav_pos_global.vi" "ADAM Positions Ch names"() -> (w652:string[])
                n206 = for {
                  tunnel: w654 -> [w667]
                  tunnel: w653 -> [w666]
                  tunnel: w652 -> [w663]
                  tunnel: T8 {"Channel Name"="", "New Value"=0.0} ("Update Scan Value Cluster") -> [w662]
                  tunnel: w646 -> [w661] mode=indexing
                  shift-right: [w657] -> w649
                  shift-left: T8[] [] -> [w658]
                  i -> [w669]
                  n207 = Format Into String(format string="%d", initial string=w667, w669) -> (resulting string=w665:string)  [unwired: 1 in, 1 out]
                  n208 = Search 1D Array(1D array=w666, element=w665) -> (index of element=w664:i32)  [unwired: 1 in]
                  n209 = Index Array(array=w663, index=w664) -> (element=w660:string)
                  n210 = Empty String/Path?(string/path=w660) -> (empty?=w659:bool)
                  n211 = case shown="False" w659 {
                    tunnel: w662 -> [w675 _]
                    tunnel: w660 -> [w674 _]
                    tunnel: w661 -> [w673 _]
                    tunnel: w658 -> [w672 w676]
                    tunnel: [w671 w676] -> w657
                    frame False {
                      n212 = Bundle By Name(cluster=w675, "Channel Name"=w674, "New Value"=w673) -> (w670:T8)
                      n213 = Build Array (concatenate)(w672, w670) -> (w671:T8[])
                    }
                    frame True {
                    }
                  }
                }
                n214 = Array Size(array=w649) -> (size(s)=w647:i32)
                n215 = Greater Than 0?(x=w647) -> (x > 0?=w648:bool)
                n216 = case shown="False" w648 {
                  tunnel: w649 -> [_ w655]
                  frame False {
                  }
                  frame True {
                    n217 = call "Read_Write_Local_table.vi"("Mode"=Global_mode."Write Global to File", "Ch Values in"=w655) -> ()  [unwired: 1 in, 3 out]
                  }
                }
              }
            }
          }
          frame "Run VI" {
          }
        }
        n218 = global write "Trav_pos_global.vi" "Traverse position"(w624) -> ()
        n219 = global write "Trav_pos_global.vi" "Live Position"(w624) -> ()
      }
      frame "Tidy up" {
        w677 = User_Specific_mode."Run VI" ("Simulate/Run")
        n220 = case shown="\"Move traverse\"" w682 {
          tunnel: w688 -> [w702 w769]
          tunnel: w687 -> [w703 w768]
          tunnel: w683 -> [w701 _]
          tunnel: [w700 w768] -> w686
          tunnel: w681 -> [w696 _]
          tunnel: w680 -> [w699 _]
          tunnel: w679 -> [w695 _]
          tunnel: w678 -> [w698 _]
          tunnel: w677 -> [w697 _]
          frame "Move traverse" {
            n221 = Equal?(x=w695, y=w697) -> (x = y?=w694:bool)
            n222 = And(x=w698, y=w694) -> (x .and. y?=w693:bool)
            n223 = case shown="True" w693 {
              tunnel: w703 -> [w708 w745]
              tunnel: w702 -> [w707 w748]
              tunnel: w701 -> [w706 _]
              tunnel: [w705 w743] -> w700
              tunnel: w699 -> [_ w742]
              tunnel: w696 -> [_ w739]
              frame False {
                n224 = Empty String/Path?(string/path=w708) -> (empty?=w704:bool)
                n225 = case shown="True" w704 {
                  tunnel: w707 -> [_ w713]
                  tunnel: w706 -> [_ w712]
                  tunnel: w708 -> [w709 w711]
                  tunnel: [w709 w710] -> w705
                  frame False {
                  }
                  frame True {
                    n226 = for {
                      tunnel: w713 -> [w716] mode=indexing
                      tunnel: w712 -> [w717] mode=indexing
                      shift-right: [w714] -> w710
                      shift-left: w711 -> [w715]
                      i -> [w720]
                      w722 = 10.0  # ±
                      n227 = case shown="0, Default" w720 {
                        tunnel: ["X" "Y" "Z"] -> w718
                        frame 0, Default {
                        }
                        frame 1 {
                        }
                        frame 2 {
                        }
                      }
                      n228 = call "In_Range_check.vi"("±"=w722, "Mode"=In_Range."±", "Value"=w717, "Setpoint"=w716) -> ("In Range"=w719:bool)  [unwired: 1 in, 2 out]
                      n229 = case shown="False" w719 {
                        tunnel: w718 -> [w729 _]
                        tunnel: w717 -> [w728 _]
                        tunnel: w716 -> [w727 _]
                        tunnel: w715 -> [w724 w730]
                        tunnel: [w725 w730] -> w714
                        frame False {
                          n230 = Format Into String(format string="For %s Axis Dem Pos = %.1f Achieved Pos = %.1f mm" ("Format String"), w729, w728, w727) -> (resulting string=w723:string)  [unwired: 2 in, 1 out]
                          n231 = Concatenate Strings(w724, w723) -> (w725:string)
                        }
                        frame True {
                        }
                      }
                    }
                  }
                }
              }
              frame True {
                n232 = local read "Position"() -> (w734:sgl[])
                n233 = case shown="\"Don't Home\"" w739 {
                  tunnel: [0 ("index") 0 ("index") 0 ("index") 1 ("index") 1 ("index") 2 ("index") 2 ("index")] -> w738
                  tunnel: ["-X" "+X" "-X" "+Y" "-Y" "+Z" "-Z"] -> w737
                  frame "Don't Home" {
                  }
                  frame "Home  +X" {
                  }
                  frame "Home  -X" {
                  }
                  frame "Home  +Y" {
                  }
                  frame "Home  -Y" {
                  }
                  frame "Home  +Z" {
                  }
                  frame "Home  -Z" {
                  }
                }
                n234 = Index Array(array=w748, index=w738) -> (element=w736:sgl)
                n235 = Index Array(array=w734, index=w738) -> (element=w735:sgl)
                n236 = Subtract(x=w736, y=w735) -> (x-y=w741:sgl)
                n237 = Multiply(x=0.995, y=w742) -> (x*y=w746:dbl)
                n238 = Absolute Value(x=w741) -> (abs(x)=w740:sgl)
                n239 = Less?(x=w740, y=w746) -> (x < y?=w744:bool)
                n240 = case shown="False" w744 {
                  tunnel: w745 -> [w766 w767]
                  tunnel: [w765 w767] -> w743
                  tunnel: w737 -> [w763 _]
                  frame False {
                    n241 = Concatenate Strings(w766, w763, " home has not been found.") -> (w765:string)
                  }
                  frame True {
                  }
                }
              }
            }
          }
          frame "Read traverse position", Default {
            n242 = local write "Position"(w769) -> ()
          }
        }
        n243 = local write "Currently on Point"(-1 ("Row Number")) -> ()
        n244 = local write "Simulate/Run"(w677) -> ()
      }
      frame "End" {
        n245 = case shown="\"Check VI only\", Default" w776 {
          tunnel: w775 -> [_ w788]
          tunnel: w774 -> [_ w785]
          tunnel: w773 -> [_ w784]
          tunnel: w772 -> [_ w783]
          frame "Check VI only", Default {
          }
          frame "Run VI" {
            n246 = case shown="\"Work in Model Coordinates\"" w788 {
              tunnel: w785 -> [w789 w792]
              tunnel: [w789 w791] -> w786
              tunnel: w784 -> [_ w790]
              frame "Work in Tunnel Coordinates" {
              }
              frame "Work in Model Coordinates" {
                n247 = call "Coordinate_rotation.vi"("Model       Roll      Pitch       Yaw (deg)"=w790, "Input Position"=w792, "Mode"=T6."To Traverse Coordinates") -> ("Output Position"=w791:sgl[])  [unwired: 2 in, 1 out]
              }
            }
            n248 = call "Read-Write_Check_Pos.vi"("Position input"=w786, "Mode"=enum16{"Read", "Write"}."Write", "Traverse Name"=w783) -> ()  [unwired: 1 out]
          }
        }
        n249 = case shown="\"Teach Position\"" w771 {
          frame "Move traverse", Default {
          }
          frame "Teach Position" {
            n250 = local write "Mode"(Trav_mode."Read traverse position" ("Mode")) -> ()
          }
        }
        n251 = local write "Route Checking?"(TRUE ("Route Checking?")) -> ()
        n252 = local write "Home"(Home."Don't Home" ("Home")) -> ()
      }
    }
  }
  "Trav Position achieved" <- w8
  "Error String" <- w12
